vi "SP_SetXY.vi"(7 "XY Speed (10-100%)":dbl, 8 "error in (no error)":errorcluster, 9 "Y in um":dbl, 10 "X in um":dbl, 11 "SemiProbe in":refnum<class "SemiProbe.lvclass">) -> (0 "error out":errorcluster, 3 "SemiProbe out":refnum<class "SemiProbe.lvclass">)   [LabVIEW 2018, in "SemiProbe.lvclass"]
uses:
  SemiProbe.lvclass
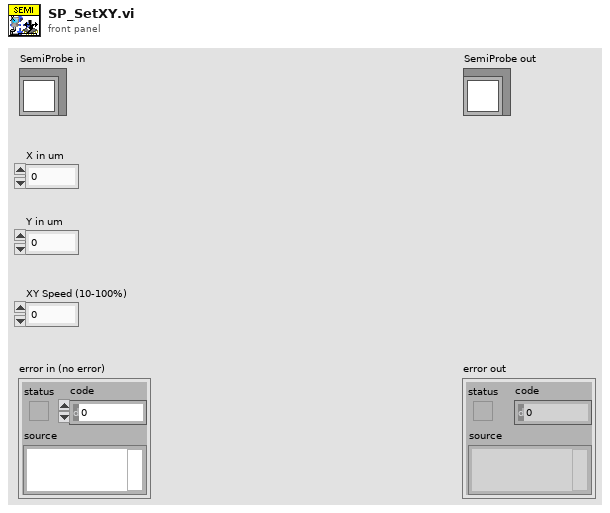
[diagram p1: front panel]
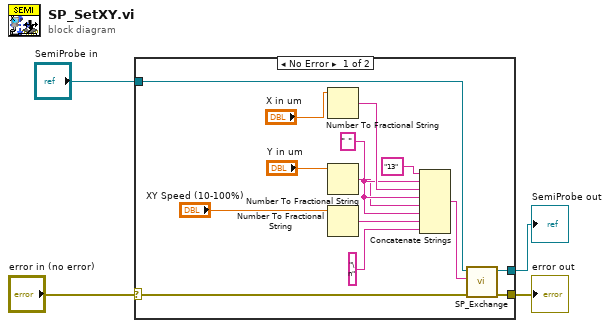
[diagram p0: block diagram]
diagram:
  n1 = case shown="No Error" "error in (no error)" {
    selector: "error in (no error)" -> [w18 w20]
    tunnel: [w17 w20] -> w3
    tunnel: [w15 w19] -> w1
    tunnel: "SemiProbe in" -> [w16 w19]
    frame No Error {
      w9 = " "
      n2 = Number To Fractional String(number="X in um") -> (F-format string=w10:string)  [unwired: 3 in]
      n3 = Number To Fractional String(number="Y in um") -> (F-format string=w8:string)  [unwired: 3 in]
      n4 = Number To Fractional String(number="XY Speed (10-100%)") -> (F-format string=w7:string)  [unwired: 3 in]
      n5 = Concatenate Strings("13", w9, w10, w9, w8, w9, w7, "\n") -> (w5:string)
      n6 = call-dynamic "SP_Exchange.vi"("error in (no error)"=w18, "command"=w5, "SemiProbe in"=w16) -> ("error out"=w17:errorcluster, "SemiProbe out"=w15:refnum<class "SemiProbe.lvclass">)  [unwired: 4 in, 3 out]
    }
    frame Error {
    }
  }
  "error out" <- w3
  "SemiProbe out" <- w1
